vi "1.隐藏饼状图.vi"(8 "error in":errorcluster, 11 "Module ID":i32=-1) -> (0 "error out":errorcluster, 3 "Module ID out":i32=-1)   [LabVIEW 2020, in "PichartInterface.lvlib"]
uses:
  PichartInterface.lvlib
  <vilib>/DD/DDToolsVIPM/PieChartInterface/PieChart.lvlibp
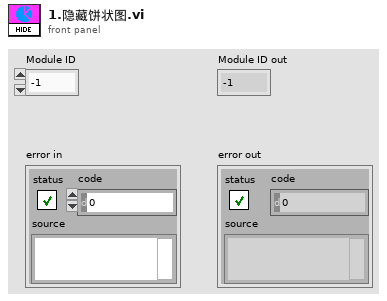
[diagram p1: front panel]
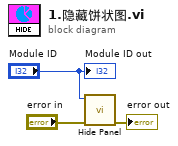
[diagram p0: block diagram]
diagram:
  n1 = call <vilib>:"Hide Panel.vi"("error in"="error in", "Module ID"="Module ID") -> ("error out"=→"error out":errorcluster)  [unwired: 9 in]
  "Module ID out" <- "Module ID"
